vi "Unflatten XML String.vi"(8 "Error In":errorcluster, 10 "XML String":string, 11 "Tree":refnum<data-value>) -> (0 "Error Out":errorcluster, 3 "Tree":refnum<data-value>)   [LabVIEW 2017, in "Tree API.lvlib" / "Tree.lvclass"]
doc: "Load the XML String specification of the Tree structure. \n\n<b>WARNING</b> This methods implements basic LV implementaion for parsing the XML. It is supported on multiple targets because it does not use the native LV DOM parser. This means it might be less optimal and not handle all XML parsing errors. Please test it extensively before using in your final design.\n\n<b>WARNING</b> When using this on an already existing Tree multiple Roots will be defined. Use the List Roots method to select the appropriate one for further use. To make sure only the contents of the XML will be represented in the resulting Tree obtain a new empty reference before calling this method."
uses:
  Tree.lvclass
  <vilib>/Utility/error.llb/Error Cluster From Error Code.vi
  <vilib>/ErrorRing/Error Ring.xnode
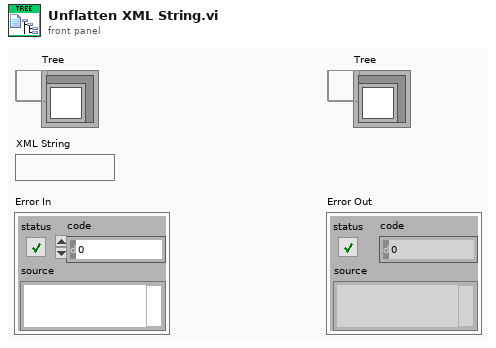
[diagram p1: front panel]
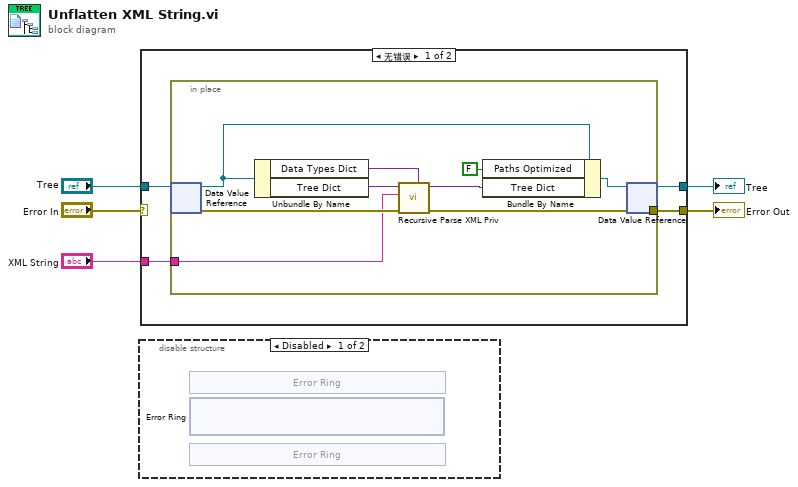
[diagram p0: block diagram]
diagram:
  n1 = disable-structure shown="Disabled" {
    frame Disabled {
      n2 = xnode "Error Ring"() -> ()  [unwired: 1 out]
      n3 = xnode "Error Ring"() -> ()  [unwired: 2 in, 1 out]
      n4 = xnode "Error Ring"() -> ()  [unwired: 1 out]
    }
    frame Enabled {
    }
  }
  n5 = case shown="无错误" "Error In" {
    selector: "Error In" -> [_ w37]
    tunnel: [w27 w37] -> w5
    tunnel: [w25 w38] -> w4
    tunnel: "Tree" -> [w26 w38]
    tunnel: "XML String" -> [w24 _]
    frame No Error {
      n6 = in-place {
        in-place-border: [w36] -> w27
        in-place-border: w24 -> [w29]
        n7 = in-place-dvr #1(w26) -> (w33:refnum<class "Tree.lvclass">, w30:errorcluster)
        n8 = Unbundle By Name(w33) -> ("Data Types Dict"=w32:variant, "Tree Dict"=w35:variant)
        n9 = call "Recursive Parse XML Priv.vi"("Data Types Dict"=w32, "Error In"=w30, "XML String"=w29, "Tree Dict"=w35) -> ("Error Out"=w36:errorcluster, "Tree Dict Out"=w34:variant)  [unwired: 5 in, 1 out]
        n10 = Bundle By Name(cluster=w33, "Paths Optimized"=FALSE, "Tree Dict"=w34) -> (w31:refnum<class "Tree.lvclass">)
        n11 = in-place-dvr #1(w31) -> (w25:refnum<data-value>)  [unwired: 1 out]
      }
    }
    frame Error {
    }
  }
  "Tree" <- w4
  "Error Out" <- w5
